vi "IECMemory.DisableCall.vi"(0 "i ref in":refnum<vi>, 3 "ms timeout (100)":i32=100, 5 "error in (no error)":errorcluster) -> (14 "i ref out":refnum<vi>, 17 "timed out":bool, 19 "error out":errorcluster)   [LabVIEW 2014, in "IECMemory.lvlib"]
doc: "When the PPG100 has finished to output its patterns, this method can be used to unregister the process and the event that has been specified with \"enable call\". What is done by this method:\n\n1) it unregisters the process and its event\n2) Go to the S0 state. In this state, the PPG100 no longer checks its state via the periodic loop\n\nThe methods \"ppg handler\" and \"enable call\" are related to this method."
uses:
  IECMemory.lvlib
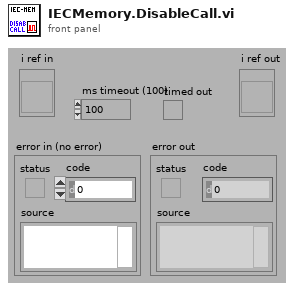
[diagram p1: front panel]
types:
  T1 = typedef "IECMemory.lvlib/IECMemory.i attribute.ctl" = cluster{"EndAddress":u32, "MemoryStatusBits":T2, "IEC Finished":bool, "Call Process":string, "Call Event":string}
  T2 = typedef "IECMemoryDriver.lvlib/Memory_Status.ctl" = bool[]
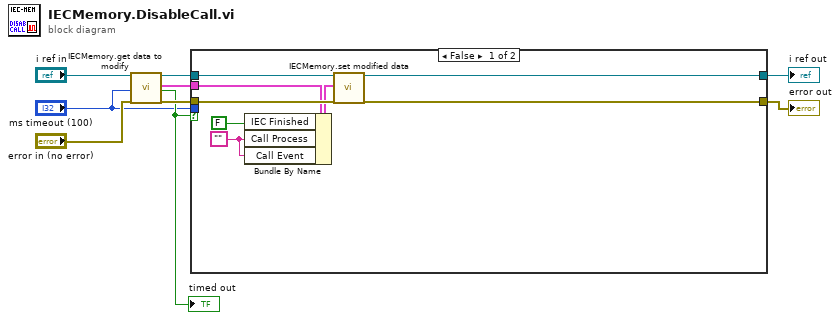
[diagram p0: block diagram]
diagram:
  n1 = call "IECMemory.get data to modify.vi"("i ref in"="i ref in", "ms timeout (10000)"="ms timeout (100)", "error in (no error)"="error in (no error)") -> ("i ref out"=w5:refnum<vi>, "i attribute"=w3:T1, "timed out"=w2:bool, "error out"=w4:errorcluster)  [unwired: 13 in]
  "timed out" <- w2
  n2 = case shown="False" w2 {
    tunnel: [w11 w18] -> w7
    tunnel: [w10 w19] -> w6
    tunnel: w5 -> [w17 w19]
    tunnel: w4 -> [w16 w18]
    tunnel: w3 -> [w14 _]
    tunnel: "ms timeout (100)" -> [_ _]
    frame False {
      w13 = ""
      n3 = Bundle By Name(cluster=w14, "IEC Finished"=FALSE ("PPG finished"), "Call Process"=w13, "Call Event"=w13) -> (w15:T1)
      n4 = call "IECMemory.set modified data.vi"("i ref in"=w17, "i attribute"=w15, "error in (no error)"=w16) -> ("i ref out"=w10:refnum<vi>, "error out"=w11:errorcluster)  [unwired: 15 in]
    }
    frame True {
    }
  }
  "error out" <- w7
  "i ref out" <- w6
